vi "参数设置页.vi"() -> ()   [LabVIEW 2016, in "斯坦道氨氮.lvlib"]
uses:
  <vilib>/Plasmionique/MB Master/MB_Master/MB_Master.lvclass
  <vilib>/ptbypt/NI_PtbyPt.lvlib
  <vilib>/Plasmionique/MB Master/MB Master.lvlib
panel:
  in  "手动模式":bool caption="手动模式(hd)"
  in  "简易流程周期设置":cluster{"switch button":bool, "设置按钮":bool}
  out "连接状态":bool
  in  "标样核查自动补测":bool caption="通讯连接"
  in  "跨度核查自动补测":bool caption="通讯连接"
  in  "零点核查自动补测":bool caption="通讯连接"
  in  "标样核查标液偏差":dbl caption="标样核查标液偏差："
  in  "跨度核查标液偏差":dbl caption="跨度核查标液偏差："
  in  "零点核查标液偏差":dbl caption="零点核查标液偏差："
  out "低量程上限":dbl caption="低量程上限：" format="%#_g mg/L"
  in  "简易流程路径":path=path "data/流程.xml"
  out "数据刷新时间":string
  in  "通讯连接":bool=TRUE
  out "MB table":enum32{"Serial", "TCP"}(tab)
  in  "请选择串口:":refnum<visa-resource-name>
  in  "波   特   率:":u32(ring)=115200 items=["115200"=115200, "9600"=9600]
  in  "协议":u16(ring)=1 caption="协         议:" items=["斯坦道协议"=1, "国标协议"=2]
  in  "IP":string="127.0.0.1"
  in  "PORT":string="1001"
  in  "通信方式选择":enum16{"串口", "TCP"}(ring)
  in  "盐度自动补偿：":bool
  out "盐度补偿值":dbl caption="盐度补偿值：" format="%#_g ppt"
  in  "刷新":bool
  in  "测量模式":T1(ring)
  in  "参数下拉列表":u16(ring)
  in  "量程下拉列表":enum16{"低量程", "高量程"}(ring)
  in  "测试流程路径":path=path "data/流程.xml"
  in  "标样核查量程模式":T2 caption="标样核查："
  in  "加标回收量程模式":T2 caption="加标回收："
  in  "跨度核查量程模式":T2 caption="跨度核查："
  in  "零点核查量程模式":T2 caption="零点核查："
  in  "水样测试量程模式":T2 caption="水样测试："
  out "稀释度":dbl caption="稀释度："
  out "阈值（高->低）":dbl caption="阈值（高->低）：" format="%#_g mg/L"
  out "阈值（低->高）":dbl caption="阈值（低->高）：" format="%#_g mg/L"
  out "量程下限":dbl caption="量程下限：" format="%#_g mg/L"
  out "高量程上限":dbl caption="高量程上限：" format="%#_g mg/L"
  out "检出限":dbl caption="检出限：" format="%#_g mg/L"
  out "曲线截距":dbl caption="曲线截距：" format="%#.6f"
  out "曲线斜率":dbl caption="曲线斜率：" format="%#.6f"
  out "二次多项式系数":dbl caption="二次多项式系数：" format="%#.6f"
  out "消解时长":dbl caption="消解时长：" format="%#_g min"
  out "消解温度":dbl caption="消解温度：" format="%#_g ℃"
  out "测量精度":u16 caption="测量精度："
  in  "标样核查标液浓度":dbl caption="标样核查标液浓度："
  in  "跨度核查标液浓度":dbl caption="跨度核查标液浓度："
  in  "零点核查标液浓度":dbl caption="零点核查标液浓度："
  in  "跨度值":dbl caption="跨度值："
  # "日质控设置"
  # "关键参数"
  # "连接设置"
  # "mg/L"
  # "mg/L"
  # "mg/L"
  # "mg/L"
  # "±"
  # "%"
  # "%"
  # "流程设置"
  # "简易流程周期设置"
  # "自动测试量程设置"
  # "设置："
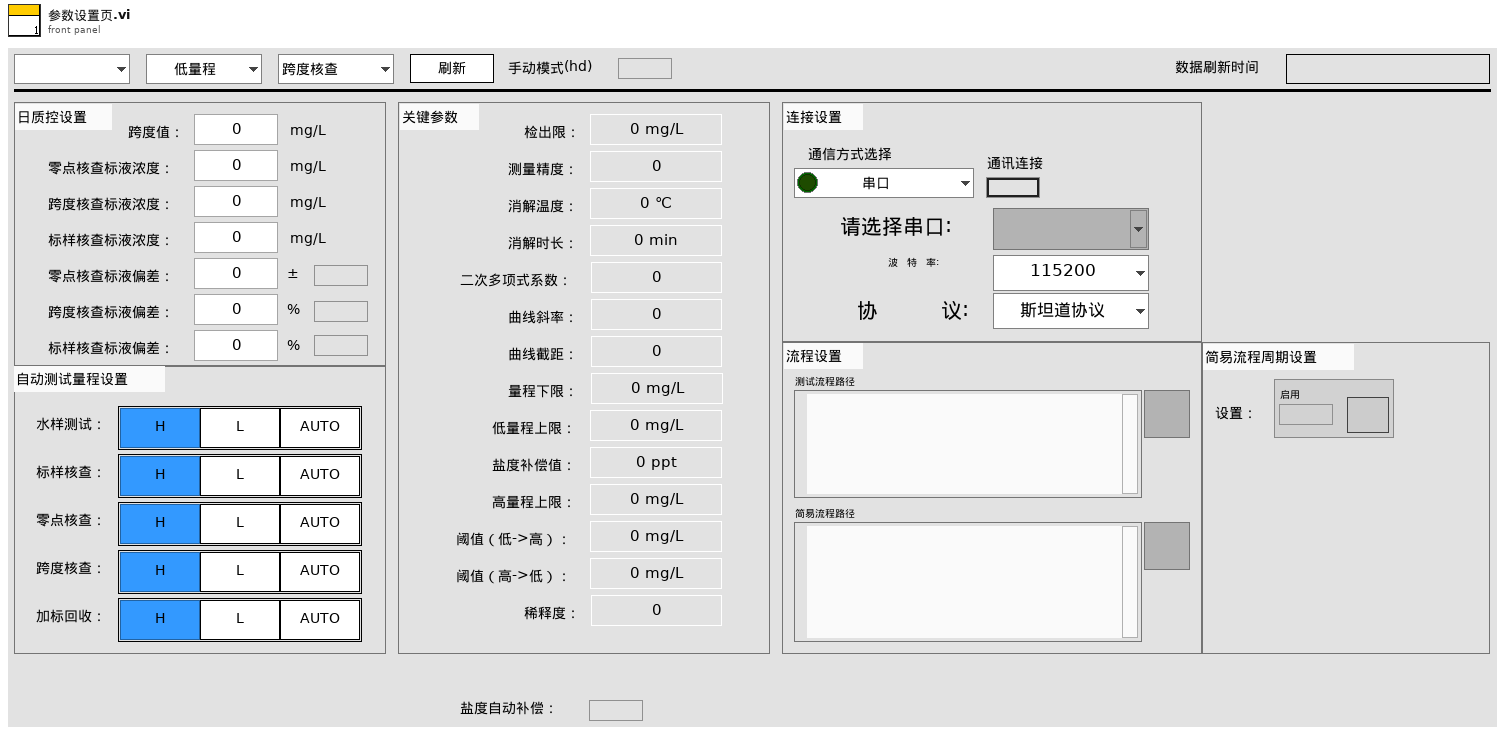
[diagram p1: front panel]
types:
  T1 = enum16{"跨度核查", "水样测量", "零点核查", "标样核查", "加标回收", "平行样测试", "空白校准", "标样校准", "空白测试"}
  T2 = typedef "斯坦道氨氮.lvlib/量程模式.ctl" = enum32{"H", "L", "AUTO"}
  T3 = typedef "Cleaning cycle.lvclass/周期项.ctl" = cluster{"时":i32, "分":i32, "频次":string, "id":i32, "参数":string, "simpleflowid":i32, "简易流程名称":string}
  T4 = cluster{"系统时间":timestamp, "工作状态":u16, "测量模式":enum16{"待机", "连续模式", "周期模式", "定点模式", "受控模式", "手动模式"}, "告警代码":u16, "故障代码":u16, "日志代码":u16, "软件版本":u16, "F0":sgl, "F1":sgl, "F2":sgl, "F3":sgl, "T":sgl, "H":sgl, "id":u16, "flowid":u16, "量程":u16, "总磷控温温度1":sgl, "营养盐控温温度2":sgl, "ADC":sgl, "结果值":sgl, "运行时间":u16, "步骤详情":string, "步骤流程":string}
  T5 = typedef "LVStringsAndValuesArrayTypeDef_U16.ctl" = cluster{"String":string, "Value":u16}[]
  T6 = enum8{"Enabled", "Disabled", "Disabled and Grayed Out"}
  T7 = cluster{"测量精度":u16, "检出限":dbl, "上限":dbl, "下限":dbl, "阈值（低->高）":dbl, "阈值（高->低）":dbl, "稀释度":dbl}
  T8 = typedef "操作日志字段定义.ctl" = cluster{"时间":timestamp, "参数":string, "日志信息":string, "流程参数":string}
  T9 = typedef "SingleStepTestV3.lvlib/SingleStepTestV3.lvclass/仪器版本.ctl" = enum16{"V3.1版", "V4版", "V3版", "V4.2版"}
  T10 = typedef "斯坦道氨氮.lvlib/V3.1版外设参数.ctl" = cluster{"泵类型":u8, "进样速度":u32, "出样速度":u32, "泵阀量":u8, "阀方向":u8, "光谱仪类型":u8, "光谱采样次数":u8, "氙灯次数":u8, "B":u16, "C":u16, "D":u16, "E":u16, "B_COD":u16, "C_COD":u16, "D_COD":u16, "E_COD":u16, "G":u16, "M":u16, "N":u16, "氨氮注射泵控温下限":sgl, "氨氮注射泵控温上限":sgl, "总氮注射泵控温下限":sgl, "总氮注射泵控温上限":sgl, "消解温度下限":sgl, "消解温度上限":sgl, "加热10s限值":sgl, "KP":sgl, "KI":sgl, "KD":sgl, "高温高压阀开阀温度":sgl, "总氮x公式0":u8, "总氮x公式1":sgl, "总氮x公式2":sgl, "总磷浊度稀释系数":sgl, "总磷浊度补偿权重1":sgl, "总磷浊度补偿权重2":sgl, "盐度系数":sgl, "氨氮补偿系数1":sgl, "氨氮补偿系数2":sgl}
  T11 = typedef "斯坦道氨氮.lvlib/V4版外设参数.ctl" = cluster{"泵类型":u8, "注射泵正常速度":u32, "注射泵慢速":u32, "阀型号":u8, "res":u8, "光谱仪类型":u8, "光谱采样次数":u8, "氙灯次数":u8, "B":u16, "C":u16, "D":u16, "E":u16, "B_COD":u16, "C_COD":u16, "D_COD":u16, "E_COD":u16, "G":u16, "M":u16, "N":u16, "降温下限":sgl, "降温上限":sgl, "恒温温度下限":sgl, "恒温温度上限":sgl, "消解温度下限":sgl, "消解温度上限":sgl, "加热10s限值":sgl, "KP":sgl, "KI":sgl, "KD":sgl, "高温高压阀开阀温度":sgl, "总氮x公式0":u8, "总氮x公式1":sgl, "总氮x公式2":sgl, "总磷浊度稀释系数":sgl, "总磷浊度补偿权重1":sgl, "总磷浊度补偿权重2":sgl, "盐度系数":sgl, "氨氮补偿系数1":sgl, "氨氮补偿系数2":sgl, "缺试剂传感器阈值":u16}
  T12 = typedef "斯坦道氨氮.lvlib/V4.2版外设参数.ctl" = cluster{"工作模式":u16, "泵类型":u16, "阀型号":u16, "注射泵进样速度":u16, "注射泵出样速度":u16, "注射泵滴定速度":u16, "res":u16, "注射泵慢速":u16, "光谱仪类型":u16, "光谱采样次数":u16, "氙灯次数":u16, "B":u16, "C":u16, "D":u16, "E":u16, "B_COD":u16, "C_COD":u16, "D_COD":u16, "E_COD":u16, "G":u16, "M":u16, "N":u16, "温度校准参数":sgl, "降温温度":sgl, "恒温温度":sgl, "消解温度":sgl, "高温高压阀开阀温度":sgl, "加热超时时间":sgl, "KP":sgl, "KI":sgl, "KD":sgl, "消解PID积分上限":sgl, "恒温PID积分上限":sgl, "PID积分下限":sgl, "缺试剂传感器阈值":u16, "滴定延时":u16, "滴定斜率阈值":sgl, "总氮x公式0":u16, "总氮x公式1":sgl, "总氮x公式2":sgl, "总磷浊度稀释系数":sgl, "总磷浊度补偿权重1":sgl, "总磷浊度补偿权重2":sgl, "盐度系数":sgl, "氨氮补偿系数1":sgl, "氨氮补偿系数2":sgl}
  T13 = typedef "斯坦道氨氮.lvlib/V3版外设参数.ctl" = cluster{"泵类型":u8, "进样速度":u32, "出样速度":u32, "泵阀量":u8, "光谱仪类型":u8, "光谱采样次数":u8, "氙灯次数":u8, "B":u16, "C":u16, "D":u16, "E":u16, "B_COD":u16, "C_COD":u16, "D_COD":u16, "E_COD":u16, "G":u16, "M":u16, "N":u16, "氨氮注射泵控温下限":sgl, "氨氮注射泵控温上限":sgl, "总氮注射泵控温下限":sgl, "总氮注射泵控温上限":sgl, "消解温度下限":sgl, "消解温度上限":sgl, "加热10s限值":sgl, "高温高压阀开阀温度":sgl, "总氮x公式0":u8, "总氮x公式1":sgl, "总氮x公式2":sgl, "总磷浊度稀释系数":sgl, "总磷浊度补偿权重1":sgl, "总磷浊度补偿权重2":sgl, "盐度系数":sgl, "氨氮补偿系数1":sgl, "氨氮补偿系数2":sgl}
  T14 = cluster{"水样测试量程模式":T2, "零点核查量程模式":T2, "跨度核查量程模式":T2, "加标回收量程模式":T2, "标样核查量程模式":T2}
  T15 = cluster{"总磷":dbl, "总氮":dbl, "氨氮":dbl, "磷酸盐":dbl, "硝氮":dbl, "亚硝氮":dbl, "硅酸盐":dbl, "硫化物":dbl, "COD":dbl, "氟化物":dbl, "CODMn":dbl}
  T16 = cluster{"总磷跨度值":dbl, "总磷零点标准液浓度":dbl, "总磷跨度标准液浓度":dbl, "总磷标准液标准浓度":dbl, "总氮跨度值":dbl, "总氮零点标准液浓度":dbl, "总氮跨度标准液浓度":dbl, "总氮标准液标准浓度":dbl, "COD跨度值":dbl, "COD零点标准液浓度":dbl, "COD跨度标准液浓度":dbl, "COD标准液标准浓度":dbl, "氨氮跨度值":dbl, "氨氮零点标准液浓度":dbl, "氨氮跨度标准液浓度":dbl, "氨氮标准液标准浓度":dbl, "磷酸盐跨度值":dbl, "磷酸盐零点标准液浓度":dbl, "磷酸盐跨度标准液浓度":dbl, "磷酸盐标准液标准浓度":dbl, "硝氮跨度值":dbl, "硝氮零点标准液浓度":dbl, "硝氮跨度标准液浓度":dbl, "硝氮标准液标准浓度":dbl, "亚硝氮跨度值":dbl, "亚硝氮零点标准液浓度":dbl, "亚硝氮跨度标准液浓度":dbl, "亚硝氮标准液标准浓度":dbl, "硫化物跨度值":dbl, "硫化物零点标准液浓度":dbl, "硫化物跨度标准液浓度":dbl, "硫化物标准液标准浓度":dbl, "硅酸盐跨度值":dbl, "硅酸盐零点标准液浓度":dbl, "硅酸盐跨度标准液浓度":dbl, "硅酸盐标准液标准浓度":dbl, "总磷零点标准液偏差":dbl, "总磷跨度标准液偏差":dbl, "总磷标准液标准偏差":dbl, "总氮零点标准液偏差":dbl, "总氮跨度标准液偏差":dbl, "总氮标准液标准偏差":dbl, "COD零点标准液偏差":dbl, "COD跨度标准液偏差":dbl, "COD标准液标准偏差":dbl, "氨氮零点标准液偏差":dbl, "氨氮跨度标准液偏差":dbl, "氨氮标准液标准偏差":dbl, "磷酸盐零点标准液偏差":dbl, "磷酸盐跨度标准液偏差":dbl, "磷酸盐标准液标准偏差":dbl, "硝氮零点标准液偏差":dbl, "硝氮跨度标准液偏差":dbl, "硝氮标准液标准偏差":dbl, "亚硝氮零点标准液偏差":dbl, "亚硝氮跨度标准液偏差":dbl, "亚硝氮标准液标准偏差":dbl, "硫化物零点标准液偏差":dbl, "硫化物跨度标准液偏差":dbl, "硫化物标准液标准偏差":dbl, "硅酸盐零点标准液偏差":dbl, "硅酸盐跨度标准液偏差":dbl, "硅酸盐标准液标准偏差":dbl, "氟化物跨度值":dbl, "氟化物零点标准液浓度":dbl, "氟化物跨度标准液浓度":dbl, "氟化物标准液标准浓度":dbl, "氟化物零点标准液偏差":dbl, "氟化物跨度标准液偏差":dbl, "氟化物标准液标准偏差":dbl, "CODMn跨度值":dbl, "CODMn零点标准液浓度":dbl, "CODMn跨度标准液浓度":dbl, "CODMn标准液标准浓度":dbl, "CODMn零点标准液偏差":dbl, "CODMn跨度标准液偏差":dbl, "CODMn标准液标准偏差":dbl}
  T17 = cluster{"测量精度":u16, "消解温度":u16, "消解时长":u16, "量程下限":sgl, "量程上限":sgl, "曲线斜率K":sgl, "曲线截距B":sgl, "标定日期":timestamp, "标液1浓度":sgl, "标液1测量过程值":sgl, "标液2浓度":sgl, "标液2测量过程值":sgl, "标液3浓度":sgl, "标液3测量过程值":sgl, "标液4浓度":sgl, "标液4测量过程值":sgl, "标液5浓度":sgl, "标液5测量过程值":sgl, "线性相关系数":sgl, "试剂余量":u32, "测量滴定值或吸光度":sgl, "空白校准时间":timestamp, "标样校准时间":timestamp, "检出限值":sgl, "校准系数":sgl, "设备系列号":string}
  T18 = cluster{"水样测试量程模式":enum16{"H", "L", "AUTO"}, "空白核查量程模式":enum16{"H", "L", "AUTO"}, "跨度核查量程模式":enum16{"H", "L", "AUTO"}, "加标回收量程模式":enum16{"H", "L", "AUTO"}, "标样核查量程模式":enum16{"H", "L", "AUTO"}}
  T19 = cluster{"水样测试量程模式":u16, "空白核查量程模式":u16, "跨度核查量程模式":u16, "加标回收量程模式":u16, "标样核查量程模式":u16}
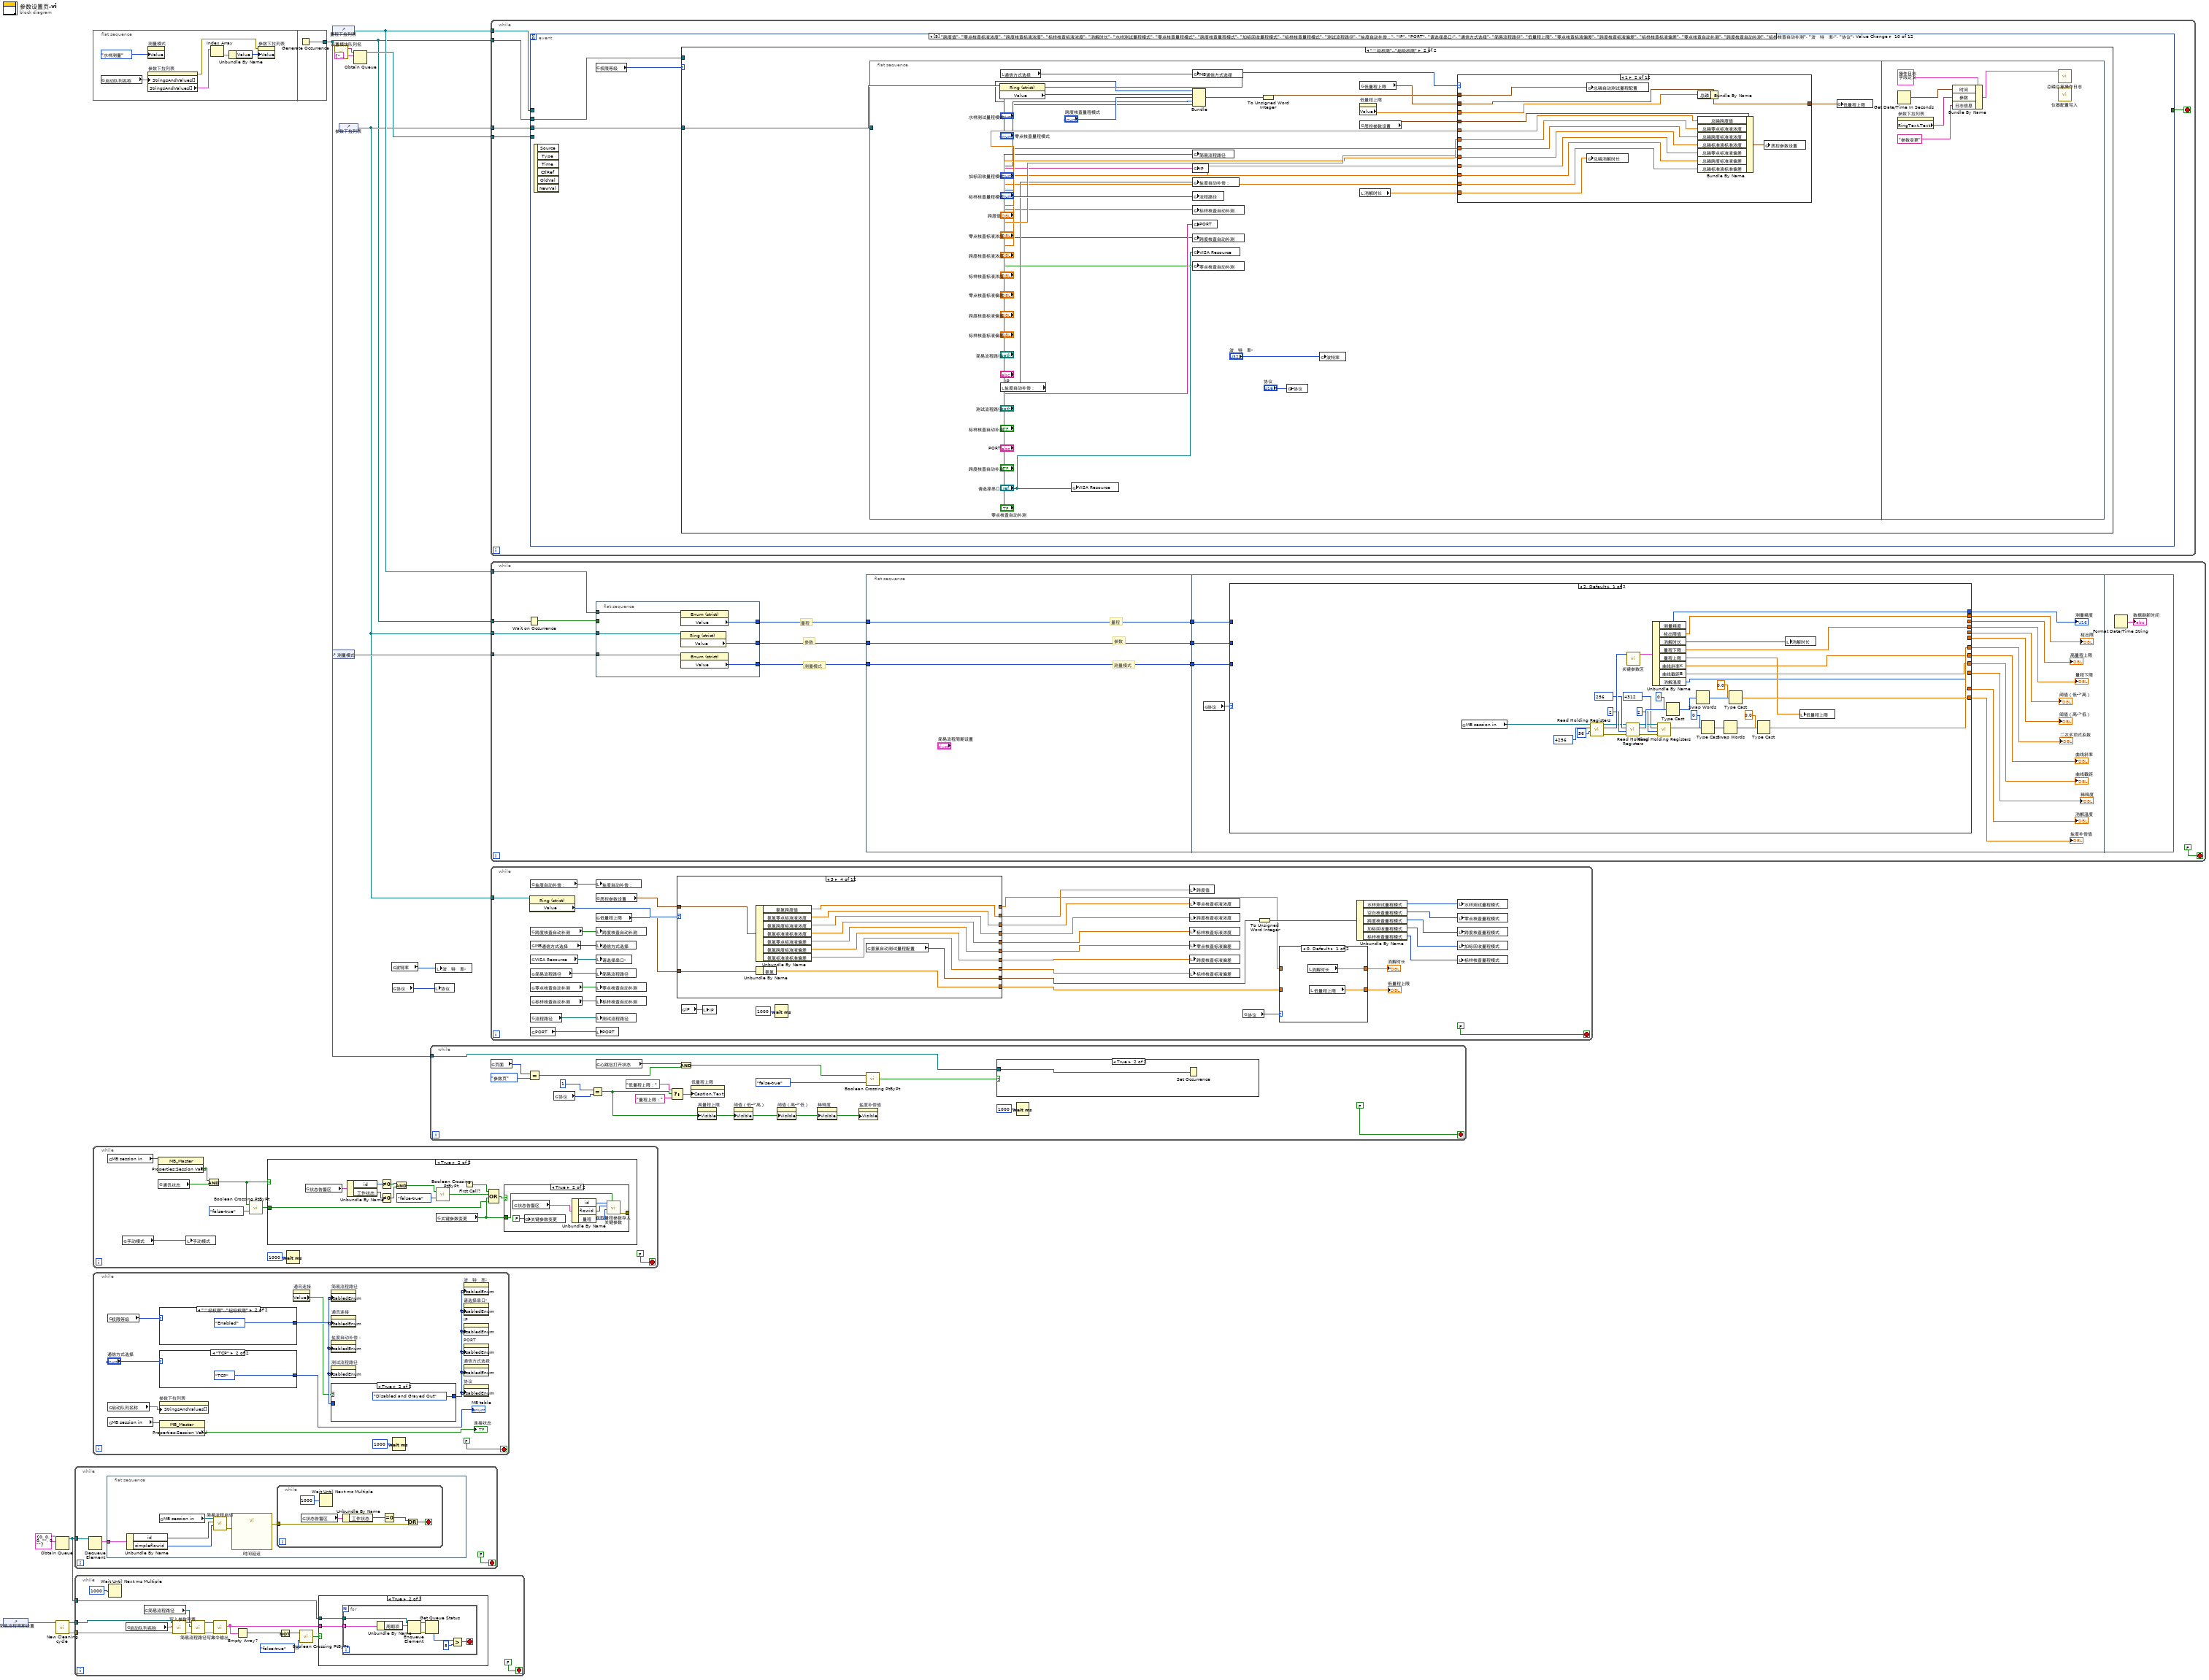
[diagram p0: block diagram]
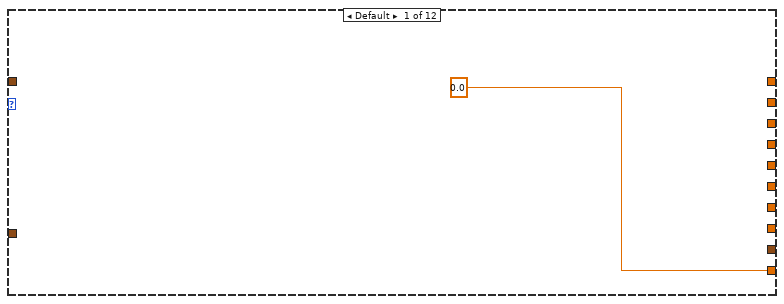
[diagram p7: hidden frame]
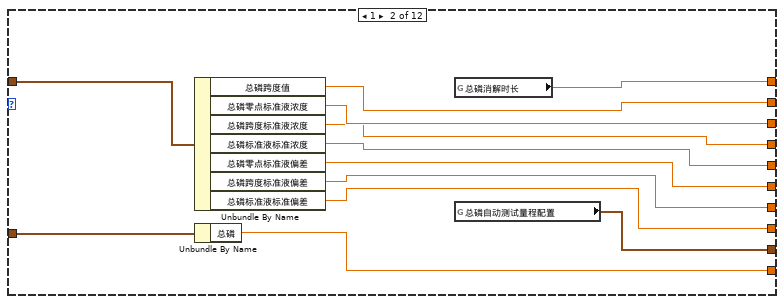
[diagram p8: hidden frame]
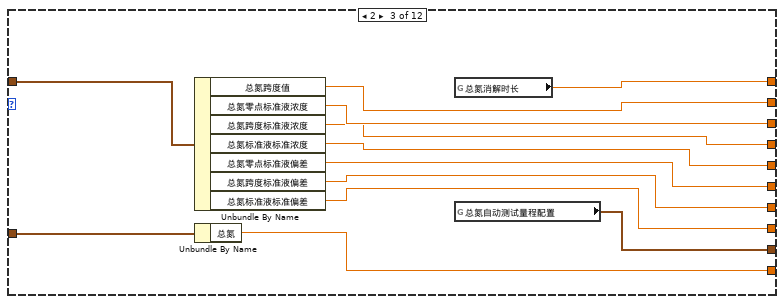
[diagram p9: hidden frame]
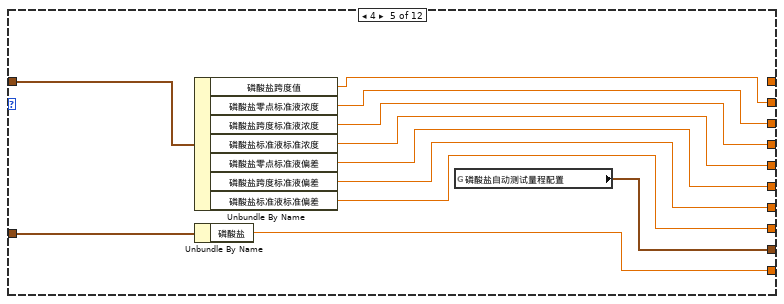
[diagram p10: hidden frame]
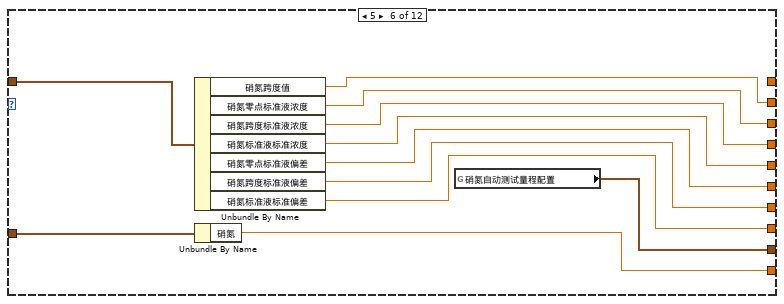
[diagram p11: hidden frame]
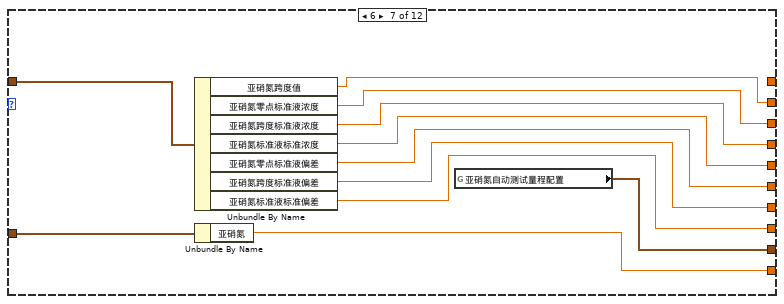
[diagram p12: hidden frame]
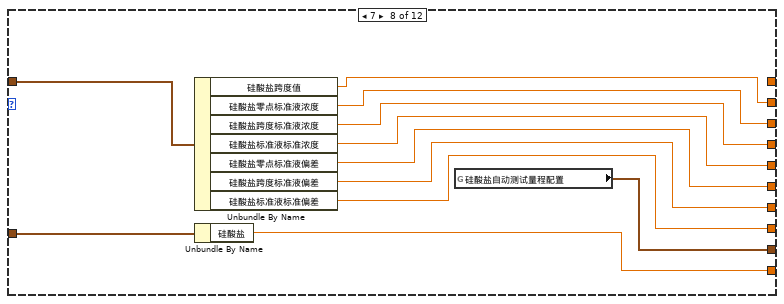
[diagram p13: hidden frame]
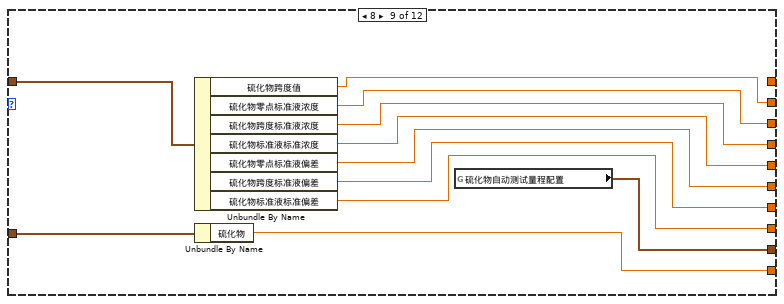
[diagram p14: hidden frame]
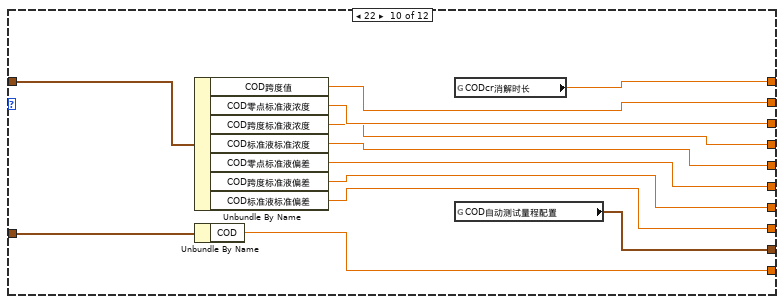
[diagram p15: hidden frame]
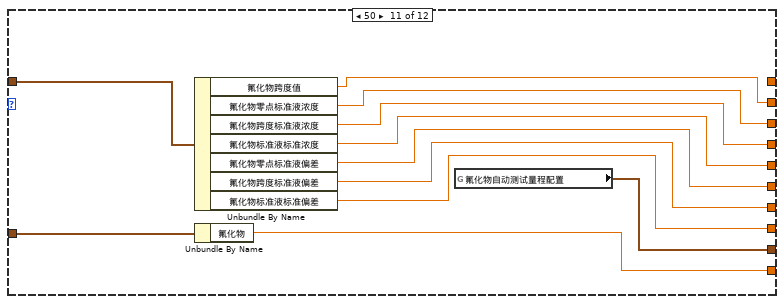
[diagram p16: hidden frame]
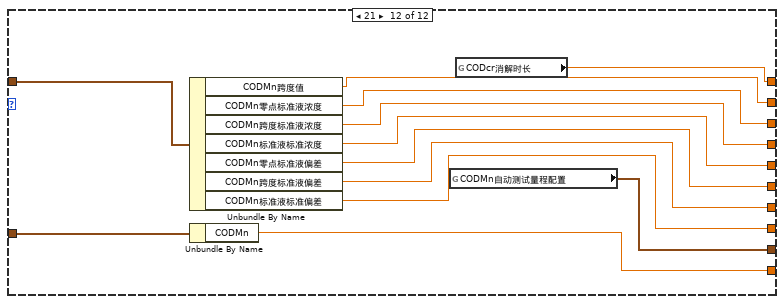
[diagram p17: hidden frame]
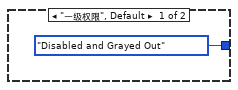
[diagram p18: hidden frame]
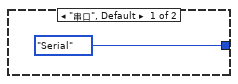
[diagram p19: hidden frame]
diagram:
  n1 = control-ref of="简易流程周期设置"() -> (w5:refnum<vi>)
  n2 = Obtain Queue(element data type=T3 {"时"=0, "分"=0, "频次"="", "id"=0, "参数"="", "simpleflowid"=0, "简易流程名称"=""} ("周期项")) -> (queue out=w3:refnum<queue>)  [unwired: 4 in, 2 out]
  n3 = call "New Cleaning cycle.vi"("Reference"=w5) -> ("error out"=w6:errorcluster, "Cleaningcycle out"=w7:refnum<class "Cleaning cycle.lvclass">)  [unwired: 9 in]
  n4 = while {
    tunnel: w3 -> [w17]
    stop <- FALSE stop-if-true
    n5 = Dequeue Element(queue=w17) -> (element=w16:T3)  [unwired: 2 in, 3 out]
    n6 = flat-sequence {
      tunnel: w16 -> [w22]
      frame #0 {
        n7 = Unbundle By Name(w22) -> ("id"=w20:i32, "simpleflowid"=w21:i32)
        n8 = global read "VAR总磷总氮全局变量.vi" "MB session in"() -> (w23:refnum<class "MB_Master.lvclass">)
        n9 = call "简易流程启动.vi"("简易流程"=w21, "参数Id"=w20, "MB session in"=w23) -> ("error out"=w19:errorcluster)  [unwired: 7 in, 1 out]
        n10 = call "时间延迟"("error in (no error)"=w19) -> ("error out"=w18:errorcluster)  [unwired: 10 in]
        n11 = while {
          tunnel: w18 -> [w25]
          stop <- w24 stop-if-true
          n12 = global read "VAR总磷总氮全局变量.vi" "状态告警区"() -> (w28:T4)
          n13 = Wait Until Next ms Multiple(millisecond multiple=u32 1000 ("毫秒倍数")) -> ()  [unwired: 1 out]
          n14 = Unbundle By Name(w28) -> ("工作状态"=w27:u16)
          n15 = Equal To 0?(x=w27) -> (x = 0?=w26:bool)
          n16 = Or(x=w26, y=w25) -> (x .or. y?=w24:bool)
        }
      }
    }
  }
  n17 = while {
    tunnel: w7 -> [w45]
    tunnel: w6 -> [w44]
    tunnel: w3 -> [w31]
    stop <- FALSE stop-if-true
    n18 = Wait Until Next ms Multiple(millisecond multiple=u32 1000 ("毫秒倍数")) -> ()  [unwired: 1 out]
    n19 = global read "model config var.vi" "启动队列名称"() -> (w41:cluster{"String":string, "Value":u16}[])
    n20 = global read "总磷总氮断电保存全局变量.vi" "简易流程路径"() -> (w40:path)
    n21 = call "写入参数列表.vi"("error in (no error)"=w44, "参数列表"=w41, "Cleaningcycle 输入"=w45) -> ("error out"=w43:errorcluster, "Cleaningcycle 输出"=w42:refnum<class "Cleaning cycle.lvclass">)  [unwired: 7 in]
    n22 = call "简易流程路径写入.vi"("error in (no error)"=w43, "简易流程路径"=w40, "Cleaningcycle 输入"=w42) -> ("error out"=w38:errorcluster, "Cleaningcycle 输出"=w39:refnum<class "Cleaning cycle.lvclass">)  [unwired: 7 in]
    n23 = call "命令输出.vi"("error in (no error)"=w38, "Cleaningcycle 输入"=w39) -> ("命令"=w33:cluster{"触发":bool, "周期项":T3}[])  [unwired: 7 in, 2 out]
    n24 = Empty Array?(array=w33) -> (empty?=w37:bool)
    n25 = Not(x=w37) -> (.not. x?=w36:bool)
    n26 = call <vilib>:"Boolean Crossing PtByPt.vi"("direction"=enum16{"either", "false-true", "true-false"}."false-true", "input"=w36) -> ("crossing"=w34:bool)  [unwired: 1 in]
    n27 = case shown="True" w34 {
      tunnel: w33 -> [_ w47]
      tunnel: w31 -> [_ w46]
      frame False {
      }
      frame True {
        n28 = for {
          tunnel: w47 -> [w55] mode=indexing
          tunnel: w46 -> [w53]
          stop <- w48 stop-if-true
          n29 = Unbundle By Name(w55) -> ("周期项"=w54:T3)
          n30 = Enqueue Element(queue=w53, element=w54) -> (queue out=w52:refnum<queue>, error out=w51:errorcluster)  [unwired: 2 in, 1 out]
          n31 = Get Queue Status(queue=w52, error in (no error)=w51) -> (# elements in queue=w50:i32)  [unwired: 1 in, 7 out]
          n32 = Greater?(x=w50, y=5) -> (0:w48:bool)
        }
      }
    }
  }
  n33 = flat-sequence {
    tunnel: [w62] -> w8
    frame #0 {
      n34 = global read "model config var.vi" "启动队列名称"() -> (w57:cluster{"String":string, "Value":u16}[])
      n35 = property on="测量模式" class="Enum (strict)"("Value"=T1."水样测量" ("测量模式")) -> ()  [unwired: 2 in, 2 out]
      n36 = property on="参数下拉列表" class="Ring (strict)"("StringsAndValues[]"=w57) -> (error out=w60:errorcluster, "StringsAndValues[]"=w58:T5)  [unwired: 2 in, 1 out]
      n37 = Index Array(array=w58) -> (element=w59:cluster{"String":string, "Value":u16})  [unwired: 1 in]
      n38 = Unbundle By Name(w59) -> ("Value"=w61:u16)
      n39 = property on="参数下拉列表" class="Ring (strict)"(error in=w60, "Value"=w61) -> ()  [unwired: 1 in, 2 out]
    }
    frame #1 {
      n40 = Generate Occurrence() -> (w62:refnum<k4>)
    }
  }
  n41 = while {
    stop <- FALSE stop-if-true
    n42 = global read "VAR总磷总氮全局变量.vi" "MB session in"() -> (w68:refnum<class "MB_Master.lvclass">)
    n43 = global read "VAR总磷总氮全局变量.vi" "手动模式"() -> (w63:bool)
    n44 = property class="MB_Master"(reference=w68) -> ("Properties:Session Valid"=w67:bool)  [unwired: 1 in, 2 out]
    n45 = global read "VAR总磷总氮全局变量.vi" "通讯状态"() -> (w70:bool)
    n46 = local write "手动模式"(w63) -> ()
    n47 = And(x=w67, y=w70) -> (x .and. y?=w65:bool)
    n48 = call <vilib>:"Boolean Crossing PtByPt.vi"("direction"=enum16{"either", "false-true", "true-false"}."false-true", "input"=w65) -> ("crossing"=w64:bool)  [unwired: 1 in]
    n49 = case shown="True" w65 {
      tunnel: w64 -> [_ w73]
      frame False {
      }
      frame True {
        n50 = global read "VAR总磷总氮全局变量.vi" "状态告警区"() -> (w83:T4)
        n51 = Unbundle By Name(w83) -> ("id"=w77:u16, "工作状态"=w82:u16)
        n52 = Not Equal To 0?(x=w77) -> (x != 0?=w78:bool)
        n53 = Not Equal To 0?(x=w82) -> (x != 0?=w79:bool)
        n54 = And(x=w78, y=w79) -> (x .and. y?=w80:bool)
        n55 = call <vilib>:"Boolean Crossing PtByPt.vi"("direction"=enum16{"either", "false-true", "true-false"}."false-true", "input"=w80) -> ("crossing"=w76:bool)  [unwired: 1 in]
        n56 = global read "VAR总磷总氮全局变量.vi" "关键参数变更"() -> (w74:bool)
        n57 = First Call?() -> (First Call?: T/F=w72:bool)
        n58 = Compound Arithmetic op=OR ("复合运算")(w72, w76, w74, w73) -> (w75:bool)
        n59 = case shown="True" w75 {
          tunnel: [_ w90] -> _
          tunnel: w74 -> [_ w85]
          frame False {
          }
          frame True {
            n60 = global read "VAR总磷总氮全局变量.vi" "状态告警区"() -> (w89:T4)
            n61 = global write "VAR总磷总氮全局变量.vi" "关键参数变更"(FALSE ("关键参数变更")) -> ()
            n62 = Unbundle By Name(w89) -> ("id"=w88:u16, "flowid"=w87:u16, "量程"=w86:u16)
            n63 = call "获取量程参数存入关键参数.vi"("关键参数变更"=w85, "量程"=w86, "flowid"=w87, "id"=w88) -> ("error out"=w90:errorcluster)  [unwired: 7 in]
          }
        }
      }
    }
    n64 = Wait (ms)(milliseconds to wait=u32 1000 ("等待时间（毫秒）")) -> ()  [unwired: 1 out]
  }
  n65 = while {
    stop <- FALSE stop-if-true
    n66 = global read "VAR总磷总氮全局变量.vi" "权限等级"() -> (w96:enum16{"一级权限", "二级权限", "三级权限", "超级权限"})
    n67 = global read "model config var.vi" "启动队列名称"() -> (w94:cluster{"String":string, "Value":u16}[])
    n68 = global read "VAR总磷总氮全局变量.vi" "MB session in"() -> (w100:refnum<class "MB_Master.lvclass">)
    n69 = case shown="\"二级权限\"..\"超级权限\"" w96 {
      tunnel: [T6."Disabled and Grayed Out" ("禁用") T6."Enabled" ("禁用")] -> w95
      frame "一级权限", Default {
      }
      frame "二级权限".."超级权限" {
      }
    }
    n70 = case shown="\"TCP\"" "通信方式选择" {
      tunnel: [enum32{"Serial", "TCP"}."Serial" ("MB table") enum32{"Serial", "TCP"}."TCP" ("MB table")] -> w98
      frame "串口", Default {
      }
      frame "TCP" {
      }
    }
    "MB table" <- w98
    n71 = property on="参数下拉列表" class="Ring (strict)"("StringsAndValues[]"=w94) -> ()  [unwired: 2 in, 2 out]
    n72 = property class="MB_Master"(reference=w100) -> ("Properties:Session Valid"=→"连接状态":bool)  [unwired: 1 in, 2 out]
    n73 = property on="通讯连接" class="Bool (strict)"() -> ("Value"=w92:bool)  [unwired: 2 in, 2 out]
    n74 = property on="简易流程路径" class="Path"("DisabledEnum"=w95) -> ()  [unwired: 2 in, 2 out]
    n75 = property on="通讯连接" class="Bool (strict)"("DisabledEnum"=w95) -> ()  [unwired: 2 in, 2 out]
    n76 = property on="盐度自动补偿：" class="Bool (strict)"("DisabledEnum"=w95) -> ()  [unwired: 2 in, 2 out]
    n77 = property on="测试流程路径" class="Path"("DisabledEnum"=w95) -> ()  [unwired: 2 in, 2 out]
    n78 = case shown="True" w92 {
      tunnel: [w106 T6."Disabled and Grayed Out" ("禁用")] -> w91
      tunnel: w95 -> [w106 _]
      frame False {
      }
      frame True {
      }
    }
    n79 = Wait (ms)(milliseconds to wait=u32 1000 ("等待时间（毫秒）")) -> ()  [unwired: 1 out]
    n80 = property on="波   特   率:" class="Ring (strict)"("DisabledEnum"=w91) -> ()  [unwired: 2 in, 2 out]
    n81 = property on="请选择串口:" class="VISAName"("DisabledEnum"=w91) -> ()  [unwired: 2 in, 2 out]
    n82 = property on="IP" class="Str"("DisabledEnum"=w91) -> ()  [unwired: 2 in, 2 out]
    n83 = property on="PORT" class="Str"("DisabledEnum"=w91) -> ()  [unwired: 2 in, 2 out]
    n84 = property on="通信方式选择" class="Enum (strict)"("DisabledEnum"=w91) -> ()  [unwired: 2 in, 2 out]
    n85 = property on="协议" class="Ring (strict)"("DisabledEnum"=w91) -> ()  [unwired: 2 in, 2 out]
  }
  n86 = control-ref of="量程下拉列表"() -> (w10:refnum<vi>)
  n87 = control-ref of="测量模式"() -> (w11:refnum<vi>)
  n88 = call "设置模块队列名.vi"() -> ("Msg"=w13:string)  [unwired: 5 in]
  n89 = control-ref of="参数下拉列表"() -> (w9:refnum<vi>)
  n90 = Obtain Queue(name (unnamed)=w13, element data type=cluster{"命令":string, "data":variant} {"命令"="", "data"=variant}) -> (queue out=w12:refnum<queue>)  [unwired: 3 in, 2 out]
  n91 = global read "总磷总氮断电保存全局变量.vi" "波特率"() -> (w1:u32)
  n92 = global read "总磷总氮断电保存全局变量.vi" "协议"() -> (w2:u16)
  n93 = while {
    tunnel: w8 -> [w120]
    stop <- FALSE stop-if-true
    n94 = global read "VAR总磷总氮全局变量.vi" "页面"() -> (w122:enum16{"主页", "参数页", "校准页"})
    n95 = Equal?(x=w122, y=enum16{"主页", "参数页", "校准页"}."参数页" ("页面")) -> (x = y?=w121:bool)
    n96 = global read "总磷总氮断电保存全局变量.vi" "协议"() -> (w113:u16)
    n97 = Equal?(x=u16 1, y=w113) -> (x = y?=w108:bool)
    n98 = global read "VAR总磷总氮全局变量.vi" "心跳包打开状态"() -> (w116:bool)
    n99 = Select(t="低量程上限：" ("标题.文本"), s=w108, f="量程上限：" ("标题.文本")) -> (s? t:f=w109:string)
    n100 = And(x=w116, y=w121) -> (x .and. y?=w117:bool)
    n101 = property on="低量程上限" class="DigNum (strict)"("Caption.Text"=w109) -> ()  [unwired: 2 in, 2 out]
    n102 = property on="高量程上限" class="DigNum (strict)"("Visible"=w108) -> ()  [unwired: 2 in, 2 out]
    n103 = property on="阈值（低->高）" class="DigNum (strict)"("Visible"=w108) -> ()  [unwired: 2 in, 2 out]
    n104 = property on="阈值（高->低）" class="DigNum (strict)"("Visible"=w108) -> ()  [unwired: 2 in, 2 out]
    n105 = property on="稀释度" class="DigNum (strict)"("Visible"=w108) -> ()  [unwired: 2 in, 2 out]
    n106 = property on="盐度补偿值" class="DigNum (strict)"("Visible"=w108) -> ()  [unwired: 2 in, 2 out]
    n107 = call <vilib>:"Boolean Crossing PtByPt.vi"("direction"=enum16{"either", "false-true", "true-false"}."false-true", "input"=w117) -> ("crossing"=w115:bool)  [unwired: 1 in]
    n108 = case shown="True" w115 {
      tunnel: w120 -> [_ w124]
      frame False {
      }
      frame True {
        n109 = Set Occurrence(w124) -> ()
      }
    }
    n110 = Wait (ms)(milliseconds to wait=u32 1000 ("等待时间（毫秒）")) -> ()  [unwired: 1 out]
  }
  n111 = local write "协议"(w2) -> ()
  n112 = local write "波   特   率:"(w1) -> ()
  n113 = while {
    tunnel: w8 -> [w128]
    tunnel: w9 -> [w127]
    tunnel: w12 -> [w126]
    tunnel: w10 -> [w125]
    stop <- w129 stop-if-true
    n114 = event shown="[9] \"跨度值\", \"零点核查标液浓度\", \"跨度核查标液浓度\", \"标样核查标液浓度\", \"消解时长\", \"水样测试量程模式\", \"零点核查量程模式\", \"跨度核查量程模式\", \"加标回收量程模式\", \"标样核查量程模式\", \"测试流程路径\", \"盐度自动补偿：\", \"IP\", \"PORT\", \"请选择串口:\", \"通信方式选择\", \"简易流程路径\", \"低量程上限\", \"零点核查标液偏差\", \"跨度核查标液偏差\", \"标样核查标液偏差\", \"零点核查自动补测\", \"跨度核查自动补测\", \"标样核查自动补测\", \"波   特   率:\", \"协议\": Value Change" {
      selector: _ -> [_ _ _ _ _ _ _ _ _ _ _ _]
      dyn-events: _ -> [_ _ _ _ _ _ _ _ _ _ _ _]
      timeout: _ -> [_ _ _ _ _ _ _ _ _ _ _ _]
      tunnel: [_ TRUE _ _ _ _ _ _ _ _ _ _] -> w129
      tunnel: w128 -> [_ _ w131 _ _ _ _ _ _ w210 _ _]
      tunnel: w127 -> [_ _ _ _ w150 _ _ _ _ w212 _ _]
      tunnel: w126 -> [_ _ _ _ _ _ _ _ _ _ w402 _]
      tunnel: w125 -> [_ _ _ _ _ _ _ _ _ _ _ _]
      event Timeout {
        n115 = event-data() -> ()  [unwired: 1 in, 3 out]
      }
      event Panel Close {
        n116 = event-data() -> ()  [unwired: 1 in, 4 out]
      }
      event "参数下拉列表", "量程下拉列表", "测量模式", "刷新": Value Change {
        n117 = event-data() -> ()  [unwired: 1 in, 6 out]
        n118 = Set Occurrence(w131) -> ()
      }
      event "跨度值", "零点核查标液浓度", "跨度核查标液浓度", "标样核查标液浓度", "消解温度", "消解时长", "检出限", "高量程上限", "量程下限", "阈值（低->高）", "阈值（高->低）", "稀释度", "低量程上限", "零点核查标液偏差", "跨度核查标液偏差", "标样核查标液偏差": Mouse Down {
        n119 = event-data() -> ("CtlRef"=w133:refnum<vi>)  [unwired: 1 in, 5 out]
        n120 = global read "VAR总磷总氮全局变量.vi" "权限等级"() -> (w132:enum16{"一级权限", "二级权限", "三级权限", "超级权限"})
        n121 = case shown="\"二级权限\"..\"超级权限\"" w132 {
          tunnel: w133 -> [_ w137]
          frame "一级权限", Default {
          }
          frame "二级权限".."超级权限" {
            n122 = property class="DigNum (strict)"(reference=w137) -> (reference out=w135:refnum<vi>, "Value"=w136:dbl)  [unwired: 1 in, 1 out]
            n123 = call "数字键盘.vi"("OldNumber"=w136) -> ("NewNumber"=w134:dbl)
            n124 = property class="DigNum (strict)"(reference=w135, "Val(Sgnl)"=w134) -> ()  [unwired: 1 in, 2 out]
          }
        }
      }
      event "测量精度", "检出限", "高量程上限", "量程下限", "阈值（低->高）", "阈值（高->低）", "稀释度": Value Change {
        n125 = event-data() -> ()  [unwired: 1 in, 6 out]
        n126 = local read "测量精度"() -> (w140:u16)
        n127 = local read "检出限"() -> (w144:dbl)
        n128 = local read "高量程上限"() -> (w146:dbl)
        n129 = local read "量程下限"() -> (w145:dbl)
        n130 = local read "阈值（低->高）"() -> (w143:dbl)
        n131 = local read "阈值（高->低）"() -> (w142:dbl)
        n132 = local read "稀释度"() -> (w141:dbl)
        n133 = property class="Ring (strict)"(reference=w150) -> ("Value"=w149:u16)  [unwired: 1 in, 2 out]
        n134 = Bundle By Name(cluster=T7 {"测量精度"=0, "检出限"=0.0, "上限"=0.0, "下限"=0.0, "阈值（低->高）"=0.0, "阈值（高->低）"=0.0, "稀释度"=0.0} ("量程参数写入"), "测量精度"=w140, "检出限"=w144, "上限"=w146, "下限"=w145, "阈值（低->高）"=w143, "阈值（高->低）"=w142, "稀释度"=w141) -> (w147:T7)
        n135 = call "量程参数写入.vi"("量程参数写入"=w147, "测量参数"=w149) -> ("error out"=w138:errorcluster)  [unwired: 8 in]
        n136 = case shown="No Error" w138 {
          tunnel: ["写入成功" "写入失败"] -> w139
          frame No Error {
            n137 = Get Date/Time In Seconds() -> (seconds since 1Jan1904=w153:timestamp)
            n138 = property on="参数下拉列表" class="Ring (strict)"() -> ("RingText.Text"=w151:string)  [unwired: 2 in, 2 out]
            n139 = Bundle By Name(cluster=T8 {"时间"=timestamp(0 s since 1904-01-01), "参数"="", "日志信息"="", "流程参数"=""} ("data in"), "时间"=w153, "参数"=w151, "日志信息"="关键参数变更") -> (w154:T8)
            n140 = call "总磷总氮操作日志.vi"("data in"=w154) -> ()  [unwired: 10 in, 1 out]
            n141 = global write "VAR总磷总氮全局变量.vi" "关键参数变更"(TRUE ("关键参数变更")) -> ()
          }
          frame Error {
          }
        }
        n142 = One Button Dialog(message=w139) -> ()  [unwired: 1 in, 1 out]
      }
      event "消解温度": Value Change {
        n143 = event-data() -> ("NewVal"=w160:dbl)  [unwired: 1 in, 5 out]
        n144 = global read "VAR总磷总氮全局变量.vi" "MB session in"() -> (w161:refnum<class "MB_Master.lvclass">)
        n145 = call "版本判断.vi"() -> ("仪器版本"=w162:T9)  [unwired: 11 in]
        n146 = case shown="\"V4.2版\"" w162 {
          tunnel: w161 -> [w170 w177 w184 w191]
          tunnel: w160 -> [w165 w173 w180 w187]
          tunnel: [w164 w171 w178 w185] -> w159
          frame "V3.1版", Default {
            n147 = call "读取V3.1外设配置.vi"("MB session in"=w170) -> ("error out"=w166:errorcluster, "外设配置"=w169:T10, "MB session out"=w168:refnum<class "MB_Master.lvclass">)  [unwired: 8 in]
            n148 = Bundle By Name(cluster=w169, "消解温度下限"=w165) -> (w167:T10)
            n149 = call "写入V3.1外设配置.vi"("error in (no error)"=w166, "外设配置"=w167, "MB session in"=w168) -> ("error out"=w164:errorcluster)  [unwired: 7 in, 1 out]
          }
          frame "V4版" {
            n150 = call "读取V4版外设配置.vi"("MB session in"=w177) -> ("error out"=w172:errorcluster, "外设配置"=w175:T11, "MB session out"=w176:refnum<class "MB_Master.lvclass">)  [unwired: 8 in]
            n151 = Bundle By Name(cluster=w175, "消解温度下限"=w173) -> (w174:T11)
            n152 = call "写入V4版外设配置.vi"("error in (no error)"=w172, "外设配置"=w174, "MB session in"=w176) -> ("error out"=w171:errorcluster)  [unwired: 7 in, 1 out]
          }
          frame "V4.2版" {
            n153 = call "读取V4.2版外设配置.vi"("MB session in"=w184) -> ("error out"=w179:errorcluster, "外设配置"=w182:T12, "MB session out"=w183:refnum<class "MB_Master.lvclass">)  [unwired: 8 in]
            n154 = Bundle By Name(cluster=w182, "消解温度"=w180) -> (w181:T12)
            n155 = call "写入V4.2版外设配置.vi"("error in (no error)"=w179, "外设配置"=w181, "MB session in"=w183) -> ("error out"=w178:errorcluster)  [unwired: 7 in, 1 out]
          }
          frame "V3版" {
            n156 = call "读取V3外设配置.vi"("MB session in"=w191) -> ("error out"=w186:errorcluster, "外设配置"=w189:T13, "MB session out"=w190:refnum<class "MB_Master.lvclass">)  [unwired: 8 in]
            n157 = Bundle By Name(cluster=w189, "消解温度下限"=w187) -> (w188:T13)
            n158 = call "写入V3外设配置.vi"("error in (no error)"=w186, "外设配置"=w188, "MB session in"=w190) -> ("error out"=w185:errorcluster)  [unwired: 7 in, 1 out]
          }
        }
        n159 = case shown="Error" w159 {
          tunnel: ["写入成功" "写入失败"] -> w163
          frame No Error {
          }
          frame Error {
          }
        }
        n160 = One Button Dialog(message=w163) -> ()  [unwired: 1 in, 1 out]
      }
      event "测量精度": Mouse Down {
        n161 = event-data() -> ("CtlRef"=w195:refnum<vi>)  [unwired: 1 in, 7 out]
        n162 = global read "VAR总磷总氮全局变量.vi" "权限等级"() -> (w194:enum16{"一级权限", "二级权限", "三级权限", "超级权限"})
        n163 = case shown="\"二级权限\"..\"超级权限\"" w194 {
          tunnel: w195 -> [_ w199]
          frame "一级权限", Default {
          }
          frame "二级权限".."超级权限" {
            n164 = property class="DigNum (strict)"(reference=w199) -> (reference out=w197:refnum<vi>, "Value"=w198:u16)  [unwired: 1 in, 1 out]
            n165 = call "数字键盘.vi"("OldNumber"=w198) -> ("NewNumber"=w196:dbl)
            n166 = property class="DigNum (strict)"(reference=w197, "Val(Sgnl)"=w196) -> ()  [unwired: 1 in, 2 out]
          }
        }
      }
      event "盐度补偿值": Mouse Down {
        n167 = event-data() -> ("CtlRef"=w201:refnum<vi>)  [unwired: 1 in, 3 out]
        n168 = global read "VAR总磷总氮全局变量.vi" "权限等级"() -> (w200:enum16{"一级权限", "二级权限", "三级权限", "超级权限"})
        n169 = case shown="\"二级权限\"..\"超级权限\"" w200 {
          tunnel: w201 -> [_ w203]
          frame "一级权限", Default {
          }
          frame "二级权限".."超级权限" {
            n170 = case shown="False" "盐度自动补偿：" {
              tunnel: w203 -> [w207 _]
              frame False {
                n171 = property class="DigNum (strict)"(reference=w207) -> (reference out=w205:refnum<vi>, "Value"=w206:dbl)  [unwired: 1 in, 1 out]
                n172 = call "数字键盘.vi"("OldNumber"=w206) -> ("NewNumber"=w204:dbl)
                n173 = property class="DigNum (strict)"(reference=w205, "Val(Sgnl)"=w204) -> ()  [unwired: 1 in, 2 out]
              }
              frame True {
              }
            }
          }
        }
      }
      event "盐度补偿值": Value Change {
        n174 = event-data() -> ("NewVal"=w208:dbl)  [unwired: 1 in, 5 out]
        n175 = global read "VAR总磷总氮全局变量.vi" "MB session in"() -> (w209:refnum<class "MB_Master.lvclass">)
        n176 = call "盐度补偿值写入.vi"("盐度补偿值"=w208, "MB session in"=w209) -> ()  [unwired: 8 in, 2 out]
      }
      event "跨度值", "零点核查标液浓度", "跨度核查标液浓度", "标样核查标液浓度", "消解时长", "测试流程路径", "盐度自动补偿：", "IP", "PORT", "请选择串口:", "通信方式选择", "简易流程路径", "低量程上限", "零点核查标液偏差", "跨度核查标液偏差", "标样核查标液偏差", "零点核查自动补测", "跨度核查自动补测", "标样核查自动补测", "波   特   率:", "协议": Value Change {
        n177 = event-data() -> ()  [unwired: 1 in, 6 out]
        n178 = global read "VAR总磷总氮全局变量.vi" "权限等级"() -> (w211:enum16{"一级权限", "二级权限", "三级权限", "超级权限"})
        n179 = case shown="\"二级权限\"..\"超级权限\"" w211 {
          tunnel: w212 -> [_ w214]
          tunnel: w210 -> [w213 _]
          frame "一级权限", Default {
            n180 = Set Occurrence(w213) -> ()
          }
          frame "二级权限".."超级权限" {
            n181 = flat-sequence {
              tunnel: w214 -> [w246]
              frame #0 {
                n182 = property class="Ring (strict)"(reference=w246) -> ("Value"=w245:u16)  [unwired: 1 in, 2 out]
                n183 = local read "通信方式选择"() -> (w229:enum16{"串口", "TCP"})
                n184 = local read "盐度自动补偿："() -> (w232:bool)
                n185 = global write "总磷总氮断电保存全局变量.vi" "VISA Resource"("请选择串口:") -> ()
                n186 = global write "总磷总氮断电保存全局变量.vi" "MB通信方式选择"(w229) -> ()
                n187 = Bundle("水样测试量程模式"="水样测试量程模式", "零点核查量程模式"="零点核查量程模式", "跨度核查量程模式"="跨度核查量程模式", "加标回收量程模式"="加标回收量程模式", "标样核查量程模式"="标样核查量程模式") -> (w234:T14)  [unwired: 1 in]
                n188 = global write "总磷总氮断电保存全局变量.vi" "简易流程路径"("简易流程路径") -> ()
                n189 = global write "总磷总氮断电保存全局变量.vi" "IP"("IP") -> ()
                n190 = global write "总磷总氮断电保存全局变量.vi" "盐度自动补偿："(w232) -> ()
                n191 = global write "总磷总氮断电保存全局变量.vi" "流程路径"("测试流程路径") -> ()
                n192 = global write "总磷总氮断电保存全局变量.vi" "标样核查自动补测"("标样核查自动补测") -> ()
                n193 = global write "总磷总氮断电保存全局变量.vi" "PORT"("PORT") -> ()
                n194 = global write "总磷总氮断电保存全局变量.vi" "跨度核查自动补测"("跨度核查自动补测") -> ()
                n195 = global write "总磷总氮断电保存全局变量.vi" "VISA Resource"("请选择串口:") -> ()
                n196 = global write "总磷总氮断电保存全局变量.vi" "零点核查自动补测"("零点核查自动补测") -> ()
                n197 = To Unsigned Word Integer(number=w234) -> (unsigned 16bit integer=w233:cluster{u16, u16, u16, u16, u16})
                n198 = global write "总磷总氮断电保存全局变量.vi" "协议"("协议") -> ()
                n199 = global write "总磷总氮断电保存全局变量.vi" "波特率"("波   特   率:") -> ()
                n200 = global read "总磷总氮断电保存全局变量.vi" "低量程上限"() -> (w226:T15)
                n201 = property on="低量程上限" class="DigNum (strict)"() -> ("Value"=w224:dbl)  [unwired: 2 in, 2 out]
                n202 = global read "总磷总氮断电保存全局变量.vi" "质控参数设置"() -> (w240:T16)
                n203 = local read "消解时长"() -> (w228:dbl)
                n204 = case shown="1" w245 {
                  tunnel: "跨度值" -> [_ w260 w274 w287 w300 w313 w326 w339 w352 w366 w380 w393]
                  tunnel: "标样核查标液浓度" -> [_ w257 w271 w284 w297 w310 w323 w336 w349 w363 w377 w390]
                  tunnel: "跨度核查标液浓度" -> [_ w258 w272 w285 w298 w311 w324 w337 w350 w364 w378 w391]
                  tunnel: "零点核查标液浓度" -> [_ w259 w273 w286 w299 w312 w325 w338 w351 w365 w379 w392]
                  tunnel: w240 -> [_ w262 w276 w289 w302 w315 w328 w341 w354 w368 w382 w395]
                  tunnel: w233 -> [_ w256 w270 w283 w296 w309 w322 w335 w348 w361 w375 w389]
                  tunnel: w228 -> [_ w255 w269 _ _ _ _ _ _ w362 w376 _]
                  tunnel: w226 -> [w248 w253 w268 w282 w295 w308 w321 w334 w347 w360 w374 w388]
                  tunnel: [w248 w252 w266 w281 w294 w307 w320 w333 w346 w359 w373 w387] -> w225
                  tunnel: w224 -> [_ w254 w267 w280 w293 w306 w319 w332 w345 w358 w372 w386]
                  tunnel: "标样核查标液偏差" -> [_ w251 w263 w277 w290 w305 w316 w329 w342 w355 w369 w383]
                  tunnel: "跨度核查标液偏差" -> [_ w250 w264 w278 w291 w304 w317 w330 w343 w356 w370 w384]
                  tunnel: "零点核查标液偏差" -> [_ w249 w265 w279 w292 w303 w318 w331 w344 w357 w371 w385]
                  frame 0, Default {
                  }
                  frame 1 {
                    n205 = global write "总磷总氮断电保存全局变量.vi" "总磷自动测试量程配置"(w256) -> ()
                    n206 = global write "总磷总氮断电保存全局变量.vi" "总磷消解时长"(w255) -> ()
                    n207 = Bundle By Name(cluster=w253, "总磷"=w254) -> (w252:T15)
                    n208 = Bundle By Name(cluster=w262, "总磷跨度值"=w260, "总磷零点标准液浓度"=w259, "总磷跨度标准液浓度"=w258, "总磷标准液标准浓度"=w257, "总磷零点标准液偏差"=w249, "总磷跨度标准液偏差"=w250, "总磷标准液标准偏差"=w251) -> (w261:T16)
                    n209 = global write "总磷总氮断电保存全局变量.vi" "质控参数设置"(w261) -> ()
                  }
                  frame 2 {
                    n210 = global write "总磷总氮断电保存全局变量.vi" "总氮自动测试量程配置"(w270) -> ()
                    n211 = global write "总磷总氮断电保存全局变量.vi" "总氮消解时长"(w269) -> ()
                    n212 = Bundle By Name(cluster=w268, "总氮"=w267) -> (w266:T15)
                    n213 = Bundle By Name(cluster=w276, "总氮跨度值"=w274, "总氮零点标准液浓度"=w273, "总氮跨度标准液浓度"=w272, "总氮标准液标准浓度"=w271, "总氮零点标准液偏差"=w265, "总氮跨度标准液偏差"=w264, "总氮标准液标准偏差"=w263) -> (w275:T16)
                    n214 = global write "总磷总氮断电保存全局变量.vi" "质控参数设置"(w275) -> ()
                  }
                  frame 3 {
                    n215 = global write "总磷总氮断电保存全局变量.vi" "氨氮自动测试量程配置"(w283) -> ()
                    n216 = Bundle By Name(cluster=w282, "氨氮"=w280) -> (w281:T15)
                    n217 = Bundle By Name(cluster=w289, "氨氮跨度值"=w287, "氨氮零点标准液浓度"=w286, "氨氮跨度标准液浓度"=w285, "氨氮标准液标准浓度"=w284, "氨氮零点标准液偏差"=w279, "氨氮跨度标准液偏差"=w278, "氨氮标准液标准偏差"=w277) -> (w288:T16)
                    n218 = global write "总磷总氮断电保存全局变量.vi" "质控参数设置"(w288) -> ()
                  }
                  frame 4 {
                    n219 = global write "总磷总氮断电保存全局变量.vi" "磷酸盐自动测试量程配置"(w296) -> ()
                    n220 = Bundle By Name(cluster=w295, "磷酸盐"=w293) -> (w294:T15)
                    n221 = Bundle By Name(cluster=w302, "磷酸盐跨度值"=w300, "磷酸盐零点标准液浓度"=w299, "磷酸盐跨度标准液浓度"=w298, "磷酸盐标准液标准浓度"=w297, "磷酸盐零点标准液偏差"=w292, "磷酸盐跨度标准液偏差"=w291, "磷酸盐标准液标准偏差"=w290) -> (w301:T16)
                    n222 = global write "总磷总氮断电保存全局变量.vi" "质控参数设置"(w301) -> ()
                  }
                  frame 5 {
                    n223 = global write "总磷总氮断电保存全局变量.vi" "硝氮自动测试量程配置"(w309) -> ()
                    n224 = Bundle By Name(cluster=w308, "硝氮"=w306) -> (w307:T15)
                    n225 = Bundle By Name(cluster=w315, "硝氮跨度值"=w313, "硝氮零点标准液浓度"=w312, "硝氮跨度标准液浓度"=w311, "硝氮标准液标准浓度"=w310, "硝氮零点标准液偏差"=w303, "硝氮跨度标准液偏差"=w304, "硝氮标准液标准偏差"=w305) -> (w314:T16)
                    n226 = global write "总磷总氮断电保存全局变量.vi" "质控参数设置"(w314) -> ()
                  }
                  frame 6 {
                    n227 = global write "总磷总氮断电保存全局变量.vi" "亚硝氮自动测试量程配置"(w322) -> ()
                    n228 = Bundle By Name(cluster=w321, "亚硝氮"=w319) -> (w320:T15)
                    n229 = Bundle By Name(cluster=w328, "亚硝氮跨度值"=w326, "亚硝氮零点标准液浓度"=w325, "亚硝氮跨度标准液浓度"=w324, "亚硝氮标准液标准浓度"=w323, "亚硝氮零点标准液偏差"=w318, "亚硝氮跨度标准液偏差"=w317, "亚硝氮标准液标准偏差"=w316) -> (w327:T16)
                    n230 = global write "总磷总氮断电保存全局变量.vi" "质控参数设置"(w327) -> ()
                  }
                  frame 7 {
                    n231 = global write "总磷总氮断电保存全局变量.vi" "硅酸盐自动测试量程配置"(w335) -> ()
                    n232 = Bundle By Name(cluster=w334, "硅酸盐"=w332) -> (w333:T15)
                    n233 = Bundle By Name(cluster=w341, "硅酸盐跨度值"=w339, "硅酸盐零点标准液浓度"=w338, "硅酸盐跨度标准液浓度"=w337, "硅酸盐标准液标准浓度"=w336, "硅酸盐零点标准液偏差"=w331, "硅酸盐跨度标准液偏差"=w330, "硅酸盐标准液标准偏差"=w329) -> (w340:T16)
                    n234 = global write "总磷总氮断电保存全局变量.vi" "质控参数设置"(w340) -> ()
                  }
                  frame 8 {
                    n235 = global write "总磷总氮断电保存全局变量.vi" "硫化物自动测试量程配置"(w348) -> ()
                    n236 = Bundle By Name(cluster=w347, "硫化物"=w345) -> (w346:T15)
                    n237 = Bundle By Name(cluster=w354, "硫化物跨度值"=w352, "硫化物零点标准液浓度"=w351, "硫化物跨度标准液浓度"=w350, "硫化物标准液标准浓度"=w349, "硫化物零点标准液偏差"=w344, "硫化物跨度标准液偏差"=w343, "硫化物标准液标准偏差"=w342) -> (w353:T16)
                    n238 = global write "总磷总氮断电保存全局变量.vi" "质控参数设置"(w353) -> ()
                  }
                  frame 22 {
                    n239 = global write "总磷总氮断电保存全局变量.vi" "COD自动测试量程配置"(w361) -> ()
                    n240 = global write "总磷总氮断电保存全局变量.vi" "CODcr消解时长"(w362) -> ()
                    n241 = Bundle By Name(cluster=w360, "COD"=w358) -> (w359:T15)
                    n242 = Bundle By Name(cluster=w368, "COD跨度值"=w366, "COD零点标准液浓度"=w365, "COD跨度标准液浓度"=w364, "COD标准液标准浓度"=w363, "COD零点标准液偏差"=w357, "COD跨度标准液偏差"=w356, "COD标准液标准偏差"=w355) -> (w367:T16)
                    n243 = global write "总磷总氮断电保存全局变量.vi" "质控参数设置"(w367) -> ()
                  }
                  frame 21 {
                    n244 = global write "总磷总氮断电保存全局变量.vi" "CODMn自动测试量程配置"(w375) -> ()
                    n245 = global write "总磷总氮断电保存全局变量.vi" "CODmn消解时长"(w376) -> ()
                    n246 = Bundle By Name(cluster=w374, "CODMn"=w372) -> (w373:T15)
                    n247 = Bundle By Name(cluster=w382, "CODMn跨度值"=w380, "CODMn零点标准液浓度"=w379, "CODMn跨度标准液浓度"=w378, "CODMn标准液标准浓度"=w377, "CODMn零点标准液偏差"=w371, "CODMn跨度标准液偏差"=w370, "CODMn标准液标准偏差"=w369) -> (w381:T16)
                    n248 = global write "总磷总氮断电保存全局变量.vi" "质控参数设置"(w381) -> ()
                  }
                  frame 50 {
                    n249 = global write "总磷总氮断电保存全局变量.vi" "氟化物自动测试量程配置"(w389) -> ()
                    n250 = Bundle By Name(cluster=w388, "氟化物"=w386) -> (w387:T15)
                    n251 = Bundle By Name(cluster=w395, "氟化物跨度值"=w393, "氟化物零点标准液浓度"=w392, "氟化物跨度标准液浓度"=w391, "氟化物标准液标准浓度"=w390, "氟化物零点标准液偏差"=w385, "氟化物跨度标准液偏差"=w384, "氟化物标准液标准偏差"=w383) -> (w394:T16)
                    n252 = global write "总磷总氮断电保存全局变量.vi" "质控参数设置"(w394) -> ()
                  }
                }
                n253 = global write "总磷总氮断电保存全局变量.vi" "低量程上限"(w225) -> ()
              }
              frame #1 {
                n254 = Get Date/Time In Seconds() -> (seconds since 1Jan1904=w398:timestamp)
                n255 = property on="参数下拉列表" class="Ring (strict)"() -> ("RingText.Text"=w396:string)  [unwired: 2 in, 2 out]
                n256 = Bundle By Name(cluster=T8 {"时间"=timestamp(0 s since 1904-01-01), "参数"="", "日志信息"="", "流程参数"=""} ("data in"), "时间"=w398, "参数"=w396, "日志信息"="参数变更") -> (w399:T8)
                n257 = call "总磷总氮操作日志.vi"("data in"=w399) -> ()  [unwired: 10 in, 1 out]
                n258 = call "仪器配置写入.vi"() -> ()  [unwired: 11 in, 1 out]
              }
            }
          }
        }
      }
      event "通讯连接": Value Change {
        n259 = event-data() -> ("NewVal"=w401:bool)  [unwired: 1 in, 5 out]
        n260 = Flush Queue(queue=w402) -> (queue out=w403:refnum<queue>)  [unwired: 1 in, 2 out]
        n261 = case shown="False" w401 {
          tunnel: w403 -> [w404 w406]
          frame False {
            n262 = Enqueue Element At Opposite End(queue=w404, element=cluster{"命令":string, "data":variant} {"命令"="停用模块", "data"=variant} ("元素")) -> ()  [unwired: 2 in, 3 out]
          }
          frame True {
            n263 = Enqueue Element At Opposite End(queue=w406, element=cluster{"命令":string, "data":variant} {"命令"="启用模块", "data"=variant} ("元素")) -> ()  [unwired: 2 in, 3 out]
          }
        }
      }
      event "手动模式": Value Change {
        n264 = event-data() -> ()  [unwired: 1 in, 6 out]
        n265 = global write "VAR总磷总氮全局变量.vi" "手动模式"("手动模式") -> ()
      }
    }
  }
  n266 = while {
    tunnel: w9 -> [w419]
    tunnel: w10 -> [w418]
    tunnel: w11 -> [w417]
    tunnel: w8 -> [w416]
    stop <- FALSE stop-if-true
    # "参数"
    # "量程"
    # "测量模式"
    n267 = Wait on Occurrence(2:w416) -> (0:w410:bool)  [unwired: 2 in]
    n268 = flat-sequence {
      tunnel: w419 -> [w426]
      tunnel: w418 -> [w425]
      tunnel: w417 -> [w424]
      tunnel: [w423] -> w413
      tunnel: [w422] -> w412
      tunnel: [w421] -> w411
      tunnel: w410 -> [_]
      frame #0 {
        n269 = property class="Enum (strict)"(reference=w425) -> ("Value"=w422:enum16{"低量程", "高量程"})  [unwired: 1 in, 2 out]
        n270 = property class="Ring (strict)"(reference=w426) -> ("Value"=w423:u16)  [unwired: 1 in, 2 out]
        n271 = property class="Enum (strict)"(reference=w424) -> ("Value"=w421:T1)  [unwired: 1 in, 2 out]
      }
    }
    n272 = flat-sequence {
      tunnel: [w429] -> w415
      tunnel: [w428] -> w414
      tunnel: w413 -> [w427]
      tunnel: w412 -> [w429]
      tunnel: w411 -> [w428]
      tunnel: [w427] -> w409
      tunnel: w415 -> [w444]
      tunnel: w414 -> [w445]
      tunnel: w409 -> [w443]
      frame #0 {
        # "参数"
        # "量程"
        # "测量模式"
      }
      frame #1 {
        n273 = global read "总磷总氮断电保存全局变量.vi" "协议"() -> (w432:u16)
        n274 = case shown="2, Default" w432 {
          tunnel: w445 -> [_ w498]
          tunnel: w444 -> [_ w497]
          tunnel: w443 -> [_ w496]
          tunnel: [w473 w494] -> w442
          tunnel: [w449 w493] -> w441
          tunnel: [_ w492] -> w440
          tunnel: [w450 w491] -> w431
          tunnel: [_ w490] -> w439
          tunnel: [_ w489] -> w438
          tunnel: [_ w488] -> w437
          tunnel: [w453 w485] -> w436
          tunnel: [w446 w484] -> w435
          tunnel: [w447 w483] -> w430
          tunnel: [w464 w480] -> w434
          tunnel: [w448 w479] -> w433
          frame 2, Default {
            n275 = global read "VAR总磷总氮全局变量.vi" "MB session in"() -> (w476:refnum<class "MB_Master.lvclass">)
            n276 = call <vilib>:"Read Holding Registers.vi"("quantity"=u16 56, "starting address"=u16 4256, "MB session in"=w476) -> ("error out"=w462:errorcluster, "Registers"=w475:u16[], "MB session out"=w470:refnum<class "MB_Master.lvclass">)  [unwired: 6 in]
            n277 = call <vilib>:"Read Holding Registers.vi"("error in (no error)"=w462, "quantity"=u16 2, "starting address"=u16 256, "MB session in"=w470) -> ("error out"=w452:errorcluster, "Registers"=w467:u16[], "MB session out"=w461:refnum<class "MB_Master.lvclass">)  [unwired: 5 in]
            n278 = call "关键参数区.vi"("数组"=w475) -> ("关键参数区"=w474:T17)  [unwired: 10 in]
            n279 = Unbundle By Name(w474) -> ("测量精度"=w473:u16, "检出限值"=w449:sgl, "消解时长"=w463:u16, "量程下限"=w450:sgl, "量程上限"=w451:sgl, "曲线斜率K"=w446:sgl, "曲线截距B"=w447:sgl, "消解温度"=w448:u16)
            n280 = call <vilib>:"Read Holding Registers.vi"("error in (no error)"=w452, "quantity"=u16 2, "starting address"=u16 4312, "MB session in"=w461) -> ("Registers"=w454:u16[])  [unwired: 5 in, 2 out]
            n281 = Type Cast(type=u32 0, x=w467) -> (*(type *) &x=w469:u32)
            n282 = Swap Words(1:w469) -> (0:w468:u32)
            n283 = Type Cast(type=u32 0, x=w454) -> (*(type *) &x=w455:u32)
            n284 = Swap Words(1:w455) -> (0:w456:u32)
            n285 = Type Cast(type=sgl 0.0, x=w468) -> (*(type *) &x=w464:sgl)
            n286 = Type Cast(type=sgl 0.0, x=w456) -> (*(type *) &x=w453:sgl)
            n287 = local write "消解时长"(w463) -> ()
            n288 = local write "低量程上限"(w451) -> ()
          }
          frame 1 {
            n289 = call "量程参数读取.vi"("测量参数"=w496) -> ("error out"=w487:errorcluster, "量程参数读取"=w495:T7)  [unwired: 9 in]
            n290 = Unbundle By Name(w495) -> ("测量精度"=w494:u16, "检出限"=w493:dbl, "上限"=w492:dbl, "下限"=w491:dbl, "阈值（低->高）"=w490:dbl, "阈值（高->低）"=w489:dbl, "稀释度"=w488:dbl)
            n291 = call "公式读取.vi"("error in (no error)"=w487, "量程"=w497, "测量模式"=w498, "测量参数"=w496) -> ("error out"=w482:errorcluster, "公式"=w486:cluster{"X^2":dbl, "X":dbl, "b":dbl})  [unwired: 6 in]
            n292 = Unbundle By Name(w486) -> ("X^2"=w485:dbl, "X"=w484:dbl, "b"=w483:dbl)
            n293 = global read "VAR总磷总氮全局变量.vi" "MB session in"() -> (w481:refnum<class "MB_Master.lvclass">)
            n294 = case shown="1..3, 21, 22" w496 {
              tunnel: [_ w501] -> w479
              tunnel: [w499 w507] -> _
              tunnel: w482 -> [w499 w502]
              tunnel: w481 -> [_ w505]
              tunnel: [_ w506] -> w480
              frame 0, Default {
              }
              frame 1..3, 21, 22 {
                n295 = call "版本判断.vi"() -> ("仪器版本"=w504:T9)  [unwired: 11 in]
                n296 = case shown="\"V3版\"" w504 {
                  tunnel: [w513 w517 w522 w528] -> w503
                  tunnel: w505 -> [w512 w518 w523 w529]
                  tunnel: [w509 w515 w520 w526] -> w501
                  tunnel: w502 -> [w511 _ _ w525]
                  tunnel: [w508 w514 w519 w524] -> w500
                  frame "V3.1版", Default {
                    n297 = call "读取V3.1外设配置.vi"("error in (no error)"=w511, "MB session in"=w512) -> ("error out"=w513:errorcluster, "外设配置"=w510:T10, "MB session out"=w508:refnum<class "MB_Master.lvclass">)  [unwired: 7 in]
                    n298 = Unbundle By Name(w510) -> ("消解温度下限"=w509:sgl)
                  }
                  frame "V4版" {
                    n299 = call "读取V4版外设配置.vi"("MB session in"=w518) -> ("error out"=w517:errorcluster, "外设配置"=w516:T11, "MB session out"=w514:refnum<class "MB_Master.lvclass">)  [unwired: 8 in]
                    n300 = Unbundle By Name(w516) -> ("消解温度下限"=w515:sgl)
                  }
                  frame "V4.2版" {
                    n301 = call "读取V4.2版外设配置.vi"("MB session in"=w523) -> ("error out"=w522:errorcluster, "外设配置"=w521:T12, "MB session out"=w519:refnum<class "MB_Master.lvclass">)  [unwired: 8 in]
                    n302 = Unbundle By Name(w521) -> ("消解温度"=w520:sgl)
                  }
                  frame "V3版" {
                    n303 = call "读取V3外设配置.vi"("error in (no error)"=w525, "MB session in"=w529) -> ("error out"=w528:errorcluster, "外设配置"=w527:T13, "MB session out"=w524:refnum<class "MB_Master.lvclass">)  [unwired: 7 in]
                    n304 = Unbundle By Name(w527) -> ("消解温度下限"=w526:sgl)
                  }
                }
                n305 = call "盐度补偿值读取.vi"("Error in"=w503, "MB session in"=w500) -> ("error out"=w507:errorcluster, "盐度补偿值"=w506:sgl)  [unwired: 7 in, 1 out]
              }
            }
          }
        }
        "测量精度" <- w442
        "检出限" <- w441
        "高量程上限" <- w440
        "量程下限" <- w431
        "阈值（低->高）" <- w439
        "阈值（高->低）" <- w438
        "稀释度" <- w437
        "二次多项式系数" <- w436
        "曲线斜率" <- w435
        "曲线截距" <- w430
        "消解温度" <- w433
        "盐度补偿值" <- w434
      }
      frame #2 {
        n306 = Format Date/Time String() -> (date/time string=→"数据刷新时间":string)  [unwired: 3 in]
      }
    }
  }
  n307 = while {
    tunnel: w9 -> [w545]
    stop <- FALSE stop-if-true
    n308 = property class="Ring (strict)"(reference=w545) -> ("Value"=w544:u16)  [unwired: 1 in, 2 out]
    n309 = global read "总磷总氮断电保存全局变量.vi" "盐度自动补偿："() -> (w559:bool)
    n310 = global read "总磷总氮断电保存全局变量.vi" "跨度核查自动补测"() -> (w536:bool)
    n311 = global read "总磷总氮断电保存全局变量.vi" "MB通信方式选择"() -> (w558:enum16{"串口", "TCP"})
    n312 = global read "总磷总氮断电保存全局变量.vi" "VISA Resource"() -> (w563:refnum<visa-resource-name>)
    n313 = global read "总磷总氮断电保存全局变量.vi" "简易流程路径"() -> (w543:path)
    n314 = global read "总磷总氮断电保存全局变量.vi" "零点核查自动补测"() -> (w538:bool)
    n315 = global read "总磷总氮断电保存全局变量.vi" "标样核查自动补测"() -> (w537:bool)
    n316 = global read "总磷总氮断电保存全局变量.vi" "流程路径"() -> (w560:path)
    n317 = global read "总磷总氮断电保存全局变量.vi" "PORT"() -> (w562:string)
    n318 = local write "盐度自动补偿："(w559) -> ()
    n319 = global read "总磷总氮断电保存全局变量.vi" "质控参数设置"() -> (w553:T16)
    n320 = global read "总磷总氮断电保存全局变量.vi" "低量程上限"() -> (w542:T15)
    n321 = local write "跨度核查自动补测"(w536) -> ()
    n322 = local write "通信方式选择"(w558) -> ()
    n323 = local write "请选择串口:"(w563) -> ()
    n324 = local write "简易流程路径"(w543) -> ()
    n325 = local write "零点核查自动补测"(w538) -> ()
    n326 = local write "标样核查自动补测"(w537) -> ()
    n327 = local write "测试流程路径"(w560) -> ()
    n328 = local write "PORT"(w562) -> ()
    n329 = case shown="3" w544 {
      tunnel: [_ w582 w594 w605 w616 w627 w638 w649 w660 w672 w683 w695] -> w552
      tunnel: [_ w581 w593 _ _ _ _ _ _ w671 _ w684] -> w532
      tunnel: w553 -> [_ w580 w592 w604 w615 w626 w637 w648 w659 w670 w682 w694]
      tunnel: [_ w579 w591 w603 w614 w625 w636 w647 w658 w669 w681 w693] -> w554
      tunnel: [_ w578 w590 w602 w613 w624 w635 w646 w657 w668 w680 w692] -> w555
      tunnel: [_ w577 w589 w601 w612 w623 w634 w645 w656 w667 w679 w691] -> w556
      tunnel: [_ w576 w588 w600 w611 w622 w633 w644 w655 w666 w678 w690] -> w557
      tunnel: w542 -> [_ w575 w587 w599 w610 w621 w632 w643 w654 w665 w677 w689]
      tunnel: [0.0 ("COD") w574 w586 w598 w609 w620 w631 w642 w653 w664 w676 w688] -> w534
      tunnel: [_ w573 w585 w597 w608 w619 w630 w641 w652 w663 w675 w687] -> w541
      tunnel: [_ w572 w584 w596 w607 w618 w629 w640 w651 w662 w674 w686] -> w540
      tunnel: [_ w571 w583 w595 w606 w617 w628 w639 w650 w661 w673 w685] -> w539
      frame Default {
      }
      frame 1 {
        n330 = Unbundle By Name(w580) -> ("总磷跨度值"=w579:dbl, "总磷零点标准液浓度"=w578:dbl, "总磷跨度标准液浓度"=w577:dbl, "总磷标准液标准浓度"=w576:dbl, "总磷零点标准液偏差"=w573:dbl, "总磷跨度标准液偏差"=w572:dbl, "总磷标准液标准偏差"=w571:dbl)
        n331 = Unbundle By Name(w575) -> ("总磷"=w574:dbl)
        n332 = global read "总磷总氮断电保存全局变量.vi" "总磷消解时长"() -> (w581:dbl)
        n333 = global read "总磷总氮断电保存全局变量.vi" "总磷自动测试量程配置"() -> (w582:T18)
      }
      frame 2 {
        n334 = Unbundle By Name(w592) -> ("总氮跨度值"=w591:dbl, "总氮零点标准液浓度"=w590:dbl, "总氮跨度标准液浓度"=w589:dbl, "总氮标准液标准浓度"=w588:dbl, "总氮零点标准液偏差"=w585:dbl, "总氮跨度标准液偏差"=w584:dbl, "总氮标准液标准偏差"=w583:dbl)
        n335 = Unbundle By Name(w587) -> ("总氮"=w586:dbl)
        n336 = global read "总磷总氮断电保存全局变量.vi" "总氮消解时长"() -> (w593:dbl)
        n337 = global read "总磷总氮断电保存全局变量.vi" "总氮自动测试量程配置"() -> (w594:T18)
      }
      frame 3 {
        n338 = Unbundle By Name(w604) -> ("氨氮跨度值"=w603:dbl, "氨氮零点标准液浓度"=w602:dbl, "氨氮跨度标准液浓度"=w601:dbl, "氨氮标准液标准浓度"=w600:dbl, "氨氮零点标准液偏差"=w597:dbl, "氨氮跨度标准液偏差"=w596:dbl, "氨氮标准液标准偏差"=w595:dbl)
        n339 = Unbundle By Name(w599) -> ("氨氮"=w598:dbl)
        n340 = global read "总磷总氮断电保存全局变量.vi" "氨氮自动测试量程配置"() -> (w605:T18)
      }
      frame 4 {
        n341 = Unbundle By Name(w615) -> ("磷酸盐跨度值"=w614:dbl, "磷酸盐零点标准液浓度"=w613:dbl, "磷酸盐跨度标准液浓度"=w612:dbl, "磷酸盐标准液标准浓度"=w611:dbl, "磷酸盐零点标准液偏差"=w608:dbl, "磷酸盐跨度标准液偏差"=w607:dbl, "磷酸盐标准液标准偏差"=w606:dbl)
        n342 = Unbundle By Name(w610) -> ("磷酸盐"=w609:dbl)
        n343 = global read "总磷总氮断电保存全局变量.vi" "磷酸盐自动测试量程配置"() -> (w616:T18)
      }
      frame 5 {
        n344 = Unbundle By Name(w626) -> ("硝氮跨度值"=w625:dbl, "硝氮零点标准液浓度"=w624:dbl, "硝氮跨度标准液浓度"=w623:dbl, "硝氮标准液标准浓度"=w622:dbl, "硝氮零点标准液偏差"=w619:dbl, "硝氮跨度标准液偏差"=w618:dbl, "硝氮标准液标准偏差"=w617:dbl)
        n345 = Unbundle By Name(w621) -> ("硝氮"=w620:dbl)
        n346 = global read "总磷总氮断电保存全局变量.vi" "硝氮自动测试量程配置"() -> (w627:T18)
      }
      frame 6 {
        n347 = Unbundle By Name(w637) -> ("亚硝氮跨度值"=w636:dbl, "亚硝氮零点标准液浓度"=w635:dbl, "亚硝氮跨度标准液浓度"=w634:dbl, "亚硝氮标准液标准浓度"=w633:dbl, "亚硝氮零点标准液偏差"=w630:dbl, "亚硝氮跨度标准液偏差"=w629:dbl, "亚硝氮标准液标准偏差"=w628:dbl)
        n348 = Unbundle By Name(w632) -> ("亚硝氮"=w631:dbl)
        n349 = global read "总磷总氮断电保存全局变量.vi" "亚硝氮自动测试量程配置"() -> (w638:T18)
      }
      frame 7 {
        n350 = Unbundle By Name(w648) -> ("硅酸盐跨度值"=w647:dbl, "硅酸盐零点标准液浓度"=w646:dbl, "硅酸盐跨度标准液浓度"=w645:dbl, "硅酸盐标准液标准浓度"=w644:dbl, "硅酸盐零点标准液偏差"=w641:dbl, "硅酸盐跨度标准液偏差"=w640:dbl, "硅酸盐标准液标准偏差"=w639:dbl)
        n351 = Unbundle By Name(w643) -> ("硅酸盐"=w642:dbl)
        n352 = global read "总磷总氮断电保存全局变量.vi" "硅酸盐自动测试量程配置"() -> (w649:T18)
      }
      frame 8 {
        n353 = Unbundle By Name(w659) -> ("硫化物跨度值"=w658:dbl, "硫化物零点标准液浓度"=w657:dbl, "硫化物跨度标准液浓度"=w656:dbl, "硫化物标准液标准浓度"=w655:dbl, "硫化物零点标准液偏差"=w652:dbl, "硫化物跨度标准液偏差"=w651:dbl, "硫化物标准液标准偏差"=w650:dbl)
        n354 = Unbundle By Name(w654) -> ("硫化物"=w653:dbl)
        n355 = global read "总磷总氮断电保存全局变量.vi" "硫化物自动测试量程配置"() -> (w660:T18)
      }
      frame 22 {
        n356 = Unbundle By Name(w670) -> ("COD跨度值"=w669:dbl, "COD零点标准液浓度"=w668:dbl, "COD跨度标准液浓度"=w667:dbl, "COD标准液标准浓度"=w666:dbl, "COD零点标准液偏差"=w663:dbl, "COD跨度标准液偏差"=w662:dbl, "COD标准液标准偏差"=w661:dbl)
        n357 = Unbundle By Name(w665) -> ("COD"=w664:dbl)
        n358 = global read "总磷总氮断电保存全局变量.vi" "CODcr消解时长"() -> (w671:dbl)
        n359 = global read "总磷总氮断电保存全局变量.vi" "COD自动测试量程配置"() -> (w672:T18)
      }
      frame 50 {
        n360 = Unbundle By Name(w682) -> ("氟化物跨度值"=w681:dbl, "氟化物零点标准液浓度"=w680:dbl, "氟化物跨度标准液浓度"=w679:dbl, "氟化物标准液标准浓度"=w678:dbl, "氟化物零点标准液偏差"=w675:dbl, "氟化物跨度标准液偏差"=w674:dbl, "氟化物标准液标准偏差"=w673:dbl)
        n361 = Unbundle By Name(w677) -> ("氟化物"=w676:dbl)
        n362 = global read "总磷总氮断电保存全局变量.vi" "氟化物自动测试量程配置"() -> (w683:T18)
      }
      frame 21 {
        n363 = Unbundle By Name(w694) -> ("CODMn跨度值"=w693:dbl, "CODMn零点标准液浓度"=w692:dbl, "CODMn跨度标准液浓度"=w691:dbl, "CODMn标准液标准浓度"=w690:dbl, "CODMn零点标准液偏差"=w687:dbl, "CODMn跨度标准液偏差"=w686:dbl, "CODMn标准液标准偏差"=w685:dbl)
        n364 = Unbundle By Name(w689) -> ("CODMn"=w688:dbl)
        n365 = global read "总磷总氮断电保存全局变量.vi" "CODMn自动测试量程配置"() -> (w695:T18)
        n366 = global read "总磷总氮断电保存全局变量.vi" "CODcr消解时长"() -> (w684:dbl)
      }
    }
    n367 = global read "总磷总氮断电保存全局变量.vi" "IP"() -> (w561:string)
    n368 = local write "IP"(w561) -> ()
    n369 = Wait (ms)(milliseconds to wait=u32 1000 ("等待时间（毫秒）")) -> ()  [unwired: 1 out]
    n370 = local write "跨度值"(w554) -> ()
    n371 = local write "零点核查标液浓度"(w555) -> ()
    n372 = local write "跨度核查标液浓度"(w556) -> ()
    n373 = local write "标样核查标液浓度"(w557) -> ()
    n374 = local write "零点核查标液偏差"(w541) -> ()
    n375 = local write "跨度核查标液偏差"(w540) -> ()
    n376 = local write "标样核查标液偏差"(w539) -> ()
    n377 = global read "总磷总氮断电保存全局变量.vi" "协议"() -> (w535:u16)
    n378 = To Unsigned Word Integer(number=w552) -> (unsigned 16bit integer=w551:T19)
    n379 = case shown="0, Default" w535 {
      tunnel: w534 -> [_ w569]
      tunnel: [w566 w569] -> w533
      tunnel: w532 -> [_ w568]
      tunnel: [w567 w568] -> w531
      frame 0, Default {
        n380 = local read "消解时长"() -> (w567:dbl)
        n381 = local read "低量程上限"() -> (w566:dbl)
      }
      frame 1 {
      }
    }
    "消解时长" <- w531
    "低量程上限" <- w533
    n382 = Unbundle By Name(w551) -> ("水样测试量程模式"=w550:u16, "空白核查量程模式"=w548:u16, "跨度核查量程模式"=w547:u16, "加标回收量程模式"=w546:u16, "标样核查量程模式"=w549:u16)
    n383 = local write "水样测试量程模式"(w550) -> ()
    n384 = local write "零点核查量程模式"(w548) -> ()
    n385 = local write "跨度核查量程模式"(w547) -> ()
    n386 = local write "加标回收量程模式"(w546) -> ()
    n387 = local write "标样核查量程模式"(w549) -> ()
  }
